vi "UpdateFPReply.vi"(1 "error in (no error)":errorcluster, 2 "Reply":string, 3 "Sent":string, 4 "method":string) -> (0 "Log":T1)   [LabVIEW 2012]
doc: "Updates log with reply from robot"
uses:
  <userlib>/ROS for LabVIEW Software/ROS/Code/Console/Servers/ServerSubs/ROSLog.ctl
  <userlib>/ROS for LabVIEW Software/ROS/Code/_ROSDefinition.vi
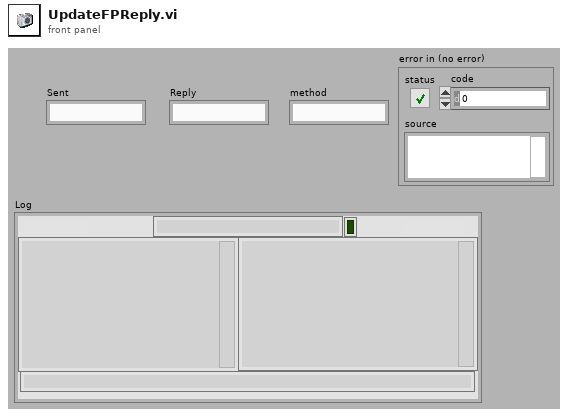
[diagram p1: front panel]
types:
  T1 = typedef "ROSLog.ctl" = cluster{"Sent":string, "Reply":string, "MethodName":string, "success":bool, "Dir1":string, "Dir2":string, "Time Stamp":string, "error":errorcluster, "Preamble":string, "Midamble":string, "Postamble":string}
  T2 = cluster{"Sent":string, "Reply":string, "method":string, bool, "element":string, "element":string, "Current Time":string, "error in (no error)":errorcluster, string, string, string}
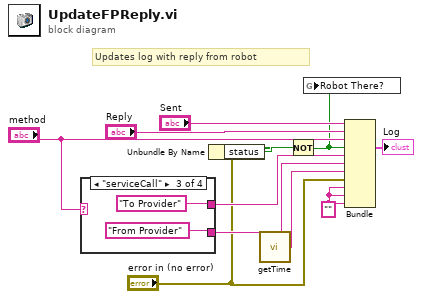
[diagram p0: block diagram]
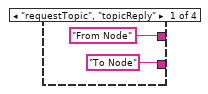
[diagram p2: hidden frame]
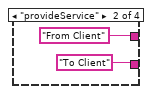
[diagram p3: hidden frame]
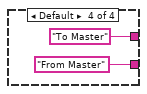
[diagram p4: hidden frame]
diagram:
  w1 = ""
  # "Updates log with reply from robot"
  n1 = case shown="\"serviceCall\"" "method" {
    tunnel: ["From Node" ("element") "From Client" ("element") "To Provider" ("element") "To Master" ("element")] -> w8
    tunnel: ["To Node" ("element") "To Client" ("element") "From Provider" ("element") "From Master" ("element")] -> w7
    frame "requestTopic", "topicReply" {
    }
    frame "provideService" {
    }
    frame "serviceCall" {
    }
    frame Default {
    }
  }
  n2 = Unbundle By Name("error in (no error)") -> ("status"=w3:bool)
  n3 = call <userlib>:"getTime.vi"() -> ("Current Time"=w6:string)  [unwired: 1 in]
  n4 = Not(x=w3) -> (.not. x?=w2:bool)
  n5 = global write "_ROSDefinition.vi" "Robot There?"(w2) -> ()
  n6 = Bundle("Sent"="Sent", "Reply"="Reply", "method"="method", w2, "element"=w8, "element"=w7, "Current Time"=w6, "error in (no error)"="error in (no error)", w1, w1, w1) -> (→"Log":T2)  [unwired: 1 in]
